vi "Request Synchronous Timestamp.vi"(6 "Ignore Past Updates? (F)":bool, 7 "Timeout In ms (-1)":i32=-1, 8 "error in (no error)":errorcluster, 9 "Type (Timestamp)":timestamp, 10 "Datum Name":string, 11 "IObserver In":refnum<class "IObserver.lvclass">) -> (0 "error out":errorcluster, 1 "timed out?":bool, 2 "Data (Timestamp)":timestamp, 4 "Publication Time":timestamp)   [LabVIEW 2015, in "IObserver.lvlib" / "IObserver.lvclass"]
doc: "<License>\nCopyright © 2017 Composed Systems, LLC | All rights reserved\nwww.composed.io\n\nAuthor: Ethan Stern <ethan.stern@composed.io>\n\nThis software is provided \"AS IS\" WITHOUT WARRANTIES, either express or implied, AND IS FOR EDUCATIONAL PURPOSES ONLY.\n</License>"
uses:
  IObserver.lvclass
  IObserver.lvclass/IObserver.ctl
  SubscriptionPolicy/OneShotSubscription/OneShotSubscription.lvclass/OneShotSubscription.ctl
  Transport/QueueTransport/QueueTransport.lvclass/QueueTransport.ctl
  IMediator/SubscriptionRequest/SubscriptionRequest.lvclass/SubscriptionRequest.ctl
  AbstractMessages/PreAddressedMsg/PreAddressedMsg.lvclass/PreAddressedMsg.ctl
  IMediator/IMediator Messages/Subscribe Msg/Subscribe Msg.lvclass/Subscribe Msg.ctl
  <vilib>/ActorFramework/Message Enqueuer/Message Enqueuer.lvclass/Message Enqueuer.ctl
  Transport/QueueTransport/New Queue Transport.vi
  IMediator/SubscriptionRequest/Pack Subscription Request.vi
  SubscriptionPolicy/OneShotSubscription/New One-Shot Subscription.vi
  IMediator/IMediator Messages/Subscribe Msg/Send Pre-Addressed Subscribe.vi
  Transport/QueueTransport/Dequeue Transport Element.vi
  <vilib>/ActorFramework/Message Enqueuer/Enqueue.vi
  AbstractMessages/PreAddressedMsg/Read Return Address.vi
  <vilib>/Utility/error.llb/Error Cluster From Error Code.vi
  <vilib>/ActorFramework/Message Priority Queue/Priority Enqueue.vi
  IMediator/ISubscriptionPolicy/Open Subscription Policy.vi
  IMediator/SubscriptionRequest/SubscriptionRequest.lvclass
  SubscriptionPolicy/OneShotSubscription/OneShotSubscription.lvclass
  Transport/QueueTransport/QueueTransport.lvclass
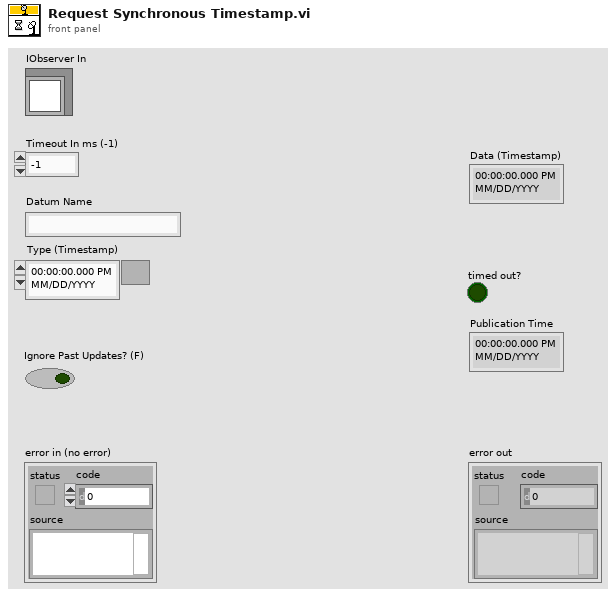
[diagram p1: front panel]
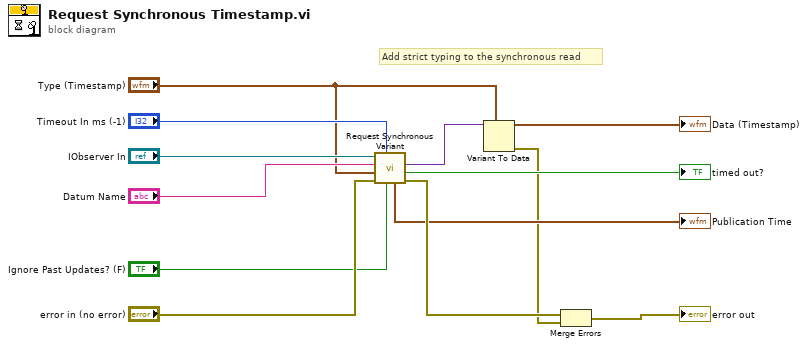
[diagram p0: block diagram]
diagram:
  # "Add strict typing to the synchronous read"
  n1 = call "Request Synchronous Variant.vi"("Ignore Past Updates? (F)"="Ignore Past Updates? (F)", "Timeout In ms (-1)"="Timeout In ms (-1)", "error in (no error)"="error in (no error)", "Type"="Type (Timestamp)", "Datum Name"="Datum Name", "IObserver In"="IObserver In") -> ("error out"=w10:errorcluster, "timed out?"=→"timed out?":bool, "Data"=w6:variant, "Publication Time"=→"Publication Time":timestamp)  [unwired: 2 in]
  n2 = Variant To Data(type="Type (Timestamp)", Variant=w6) -> (data=→"Data (Timestamp)":timestamp, error out=w1:errorcluster)  [unwired: 1 in]
  n3 = Merge Errors(w10, w1) -> (→"error out":errorcluster)
